vi "clearTelemetry.vi"(8 "error in (no error)":errorcluster, 11 "FPGATelemetry in":refnum<class "FPGATelemetry.lvclass">) -> (0 "error out":errorcluster, 3 "FPGATelemetry out":refnum<class "FPGATelemetry.lvclass">)   [LabVIEW 2015, in "FPGATelemetry.lvclass"]
uses:
  FPGATelemetry.lvclass
  FPGATelemetry.lvclass/FPGATelemetry.ctl
  <vilib>/Utility/error.llb/Error Cluster From Error Code.vi
  <vilib>/rvi/errors/niLvFpgaAdjustHostInterfaceError.vi
  <vilib>/rvi/interface/nirviMethod/nirviMethod.xnode
  <vilib>/FPGAPlugInAG/Dynamic/niLvFpga_WriteFifo_Dynamic.vi
  <vilib>/rvi/errors/niLvFpgaMergeErrorWithErrorCode.vi
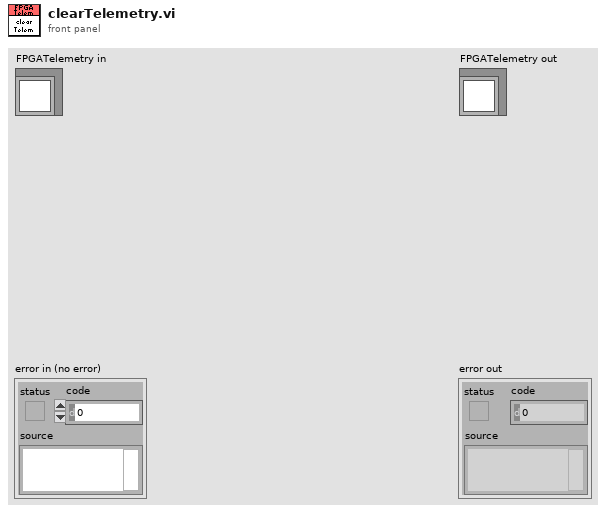
[diagram p1: front panel]
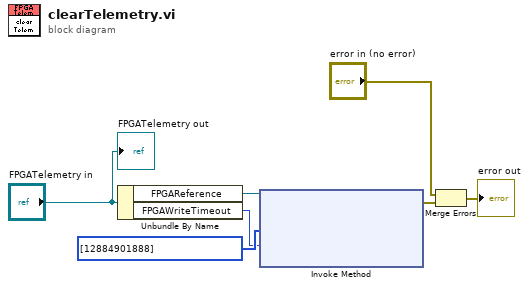
[diagram p0: block diagram]
diagram:
  n1 = Unbundle By Name("FPGATelemetry in") -> ("FPGAReference"=w7:refnum<k20>, "FPGAWriteTimeout"=w5:i32)
  n2 = xnode "Invoke Method"("FPGA VI Reference In"=w7, "Data"=u64[] [12884901888], "Timeout (ms)"=w5) -> ("error out"=w2:errorcluster)  [unwired: 1 in, 2 out]
  n3 = Merge Errors("error in (no error)", w2) -> (→"error out":errorcluster)
  "FPGATelemetry out" <- "FPGATelemetry in"
